vi "Configure Frequency Counter.vi"(5 "Enable Counter (T: Enable)":bool=TRUE, 6 "Reference Frequency (10 MHz)":dbl=10000000.0, 7 "Enable HFR (F: Disable)":bool, 8 "error in (no error)":errorcluster, 9 "Trigger Level (0.000 V)":dbl min=-3.0 max=1.8 format="%.3f", 10 "Coupling (0:AC)":u16(ring) items=["AC", "DC"], 11 "VISA resource name":refnum<visa-resource-name>) -> (0 "error out":errorcluster, 3 "VISA resource name out":refnum<visa-resource-name>)   [LabVIEW 2023, in "Siglent SDG X Series.lvlib"]
doc: "Configures and enables the built-in frequency counter."
uses:
  Siglent SDG X Series.lvlib
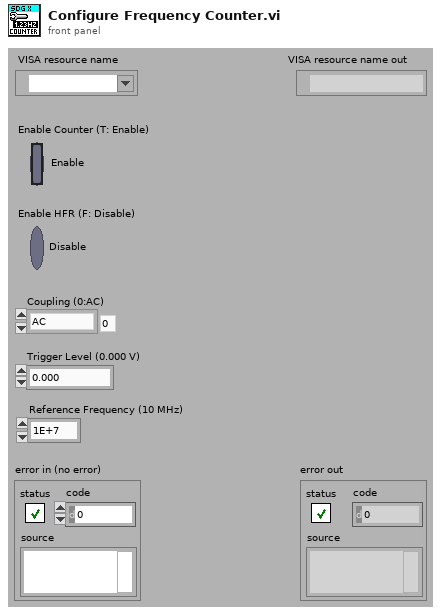
[diagram p1: front panel]
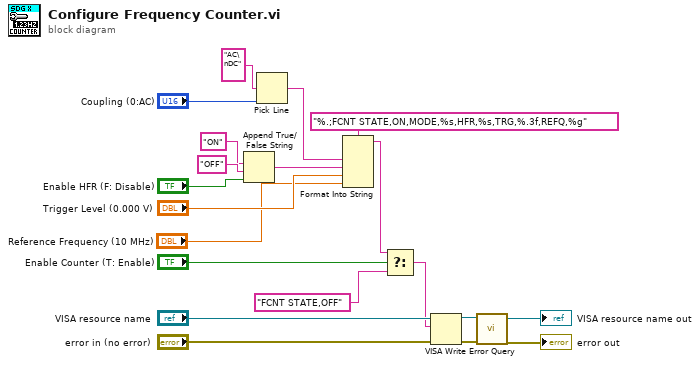
[diagram p0: block diagram]
diagram:
  n1 = Append True/False String(1:"Enable HFR (F: Disable)", 2:"OFF", 3:"ON") -> (0:w7:string)  [unwired: 1 in]
  n2 = Pick Line(multi-line string="AC\nDC", line index="Coupling (0:AC)") -> (output string=w11:string)  [unwired: 1 in]
  n3 = Format Into String(format string="%.;FCNT STATE,ON,MODE,%s,HFR,%s,TRG,%.3f,REFQ,%g", w11, w7, "Trigger Level (0.000 V)", "Reference Frequency (10 MHz)") -> (resulting string=w4:string)  [unwired: 2 in, 1 out]
  n4 = Select(t=w4, s="Enable Counter (T: Enable)", f="FCNT STATE,OFF") -> (s? t:f=w2:string)
  n5 = VISA Write(VISA resource name="VISA resource name", write buffer=w2, error in (no error)="error in (no error)") -> (VISA resource name out=w18:refnum<visa-resource-name>, error out=w17:errorcluster)  [unwired: 1 out]
  n6 = call "Error Query.vi"("error in (no error)"=w17, "VISA resource name"=w18) -> ("error out"=→"error out":errorcluster, "VISA resource name out"=→"VISA resource name out":refnum<visa-resource-name>)  [unwired: 6 in, 2 out]
